vi "关闭串口.vi"() -> ()   [LabVIEW 2017]
panel:
  in  "模拟信号串口号 2":refnum<visa-resource-name>="COM6"
  in  "模拟信号串口号":refnum<visa-resource-name>="COM6"
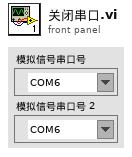
[diagram p1: front panel]
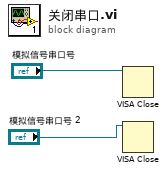
[diagram p0: block diagram]
diagram:
  n1 = VISA Close(VISA resource name="模拟信号串口号") -> ()  [unwired: 1 in, 1 out]
  n2 = VISA Close(VISA resource name="模拟信号串口号 2") -> ()  [unwired: 1 in, 1 out]
